vi "CRYDc volts out visa.vi"(10 "Volts":dbl step=0.0001 format="%.4f", 11 "COM port (0=COM1, etc.)":i32) -> (0 "error":bool)   [LabVIEW 2013]
panel:
  in  "VISA session (for class)":refnum<visa-resource-name>
  out "number":u16=28671 format="%.0x"
  out "error code":i32
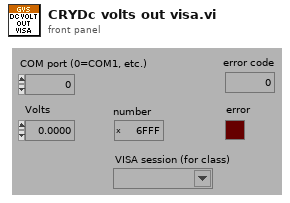
[diagram p1: front panel]
types:
  T1 = enum16{"noop", "clear DTR", "set DTR", "clear RTS", "set RTS", "set DTR protocol", "clr DTR protocol", "noop2"}
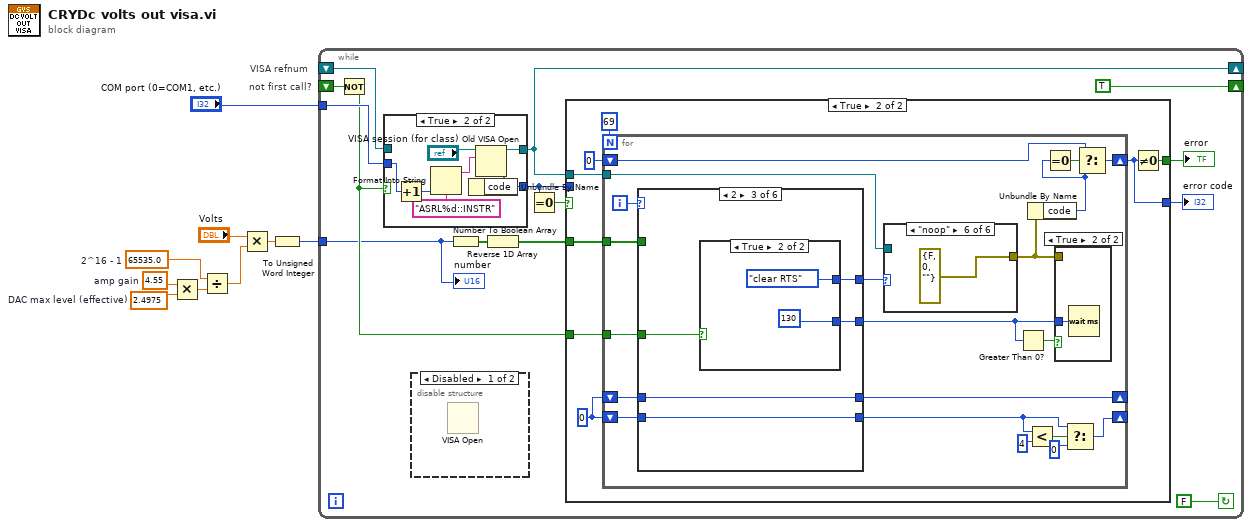
[diagram p0: block diagram]
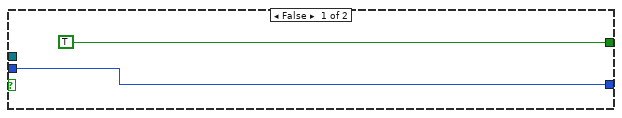
[diagram p3: hidden frame]
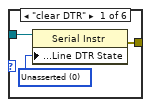
[diagram p4: hidden frame]
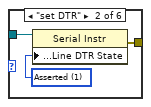
[diagram p5: hidden frame]
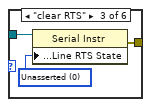
[diagram p6: hidden frame]
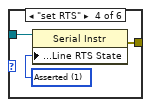
[diagram p7: hidden frame]
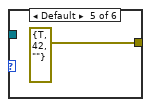
[diagram p8: hidden frame]
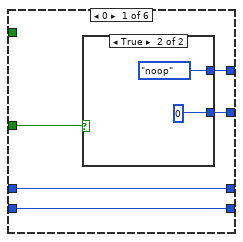
[diagram p10: hidden frame]
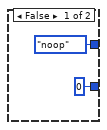
[diagram p11: hidden frame]
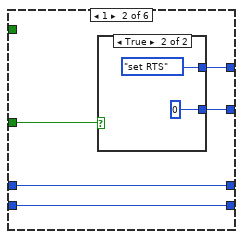
[diagram p12: hidden frame]
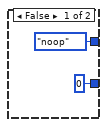
[diagram p13: hidden frame]
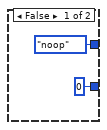
[diagram p14: hidden frame]
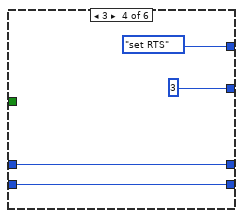
[diagram p15: hidden frame]
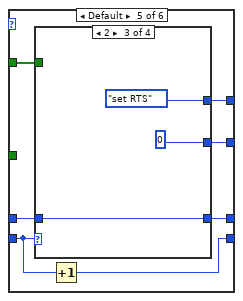
[diagram p16: hidden frame]
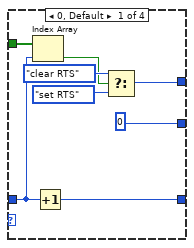
[diagram p17: hidden frame]
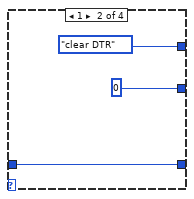
[diagram p18: hidden frame]
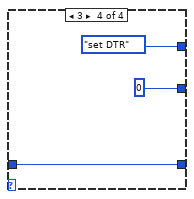
[diagram p19: hidden frame]
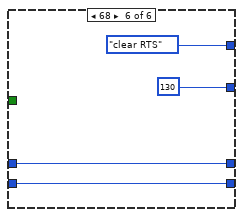
[diagram p20: hidden frame]
diagram:
  w5 = 2.4975  # DAC max level (effective)
  w7 = 65535.0  # 2^16 - 1
  w6 = 4.55  # amp gain
  # "VISA refnum"
  # "not first call?"
  n1 = Multiply(x=w6, y=w5) -> (x*y=w8:dbl)
  n2 = Divide(x=w7, y=w8) -> (x/y=w3:dbl)
  n3 = Multiply(x="Volts", y=w3) -> (x*y=w2:dbl)
  n4 = To Unsigned Word Integer(number=w2) -> (unsigned 16bit integer=w1:u16)
  n5 = while {
    tunnel: "COM port (0=COM1, etc.)" -> [w21]
    shift-right: [TRUE] -> _
    shift-left: _ -> [w19]
    tunnel: w1 -> [w17]
    shift-right: [w11] -> _
    shift-left: _ -> [w12]
    stop <- FALSE continue-if-true
    n6 = Not(x=w19) -> (.not. x?=w18:bool)
    n7 = case shown="True" w18 {
      tunnel: w21 -> [_ w135]
      tunnel: [0 ("error code") w130] -> w13
      tunnel: [w128 w132] -> w11
      tunnel: w12 -> [w128 _]
      frame False {
      }
      frame True {
        n8 = Increment(x=w135) -> (x+1=w134:i32)
        n9 = Format Into String(format string="ASRL%d::INSTR", w134) -> (resulting string=w136:string)  [unwired: 2 in, 1 out]
        n10 = Old VISA Open(10:w136, 11:"VISA session (for class)") -> (0:w131:errorcluster, 3:w132:refnum<visa-resource-name>)  [unwired: 1 in, 2 out]
        n11 = Unbundle By Name(w131) -> ("code"=w130:i32)
      }
    }
    n12 = disable-structure shown="Disabled" {
      frame Disabled {
        n13 = VISA Open() -> ()  [unwired: 5 in, 2 out]
      }
      frame Enabled {
      }
    }
    n14 = Number To Boolean Array(number=w17) -> (Boolean array=w23:bool[])
    n15 = Reverse 1D Array(array=w23) -> (reversed array=w22:bool[])
    n16 = Equal To 0?(x=w13) -> (x = 0?=w16:bool)
    n17 = case shown="True" w16 {
      tunnel: w22 -> [_ w33]
      tunnel: w18 -> [_ w30]
      tunnel: [TRUE w28] -> w15
      tunnel: [w24 w27] -> w14
      tunnel: w13 -> [w24 _]
      tunnel: w11 -> [_ w26]
      frame False {
      }
      frame True {
        w32 = 0
        n18 = for {
          N: 69 -> [_]
          tunnel: w33 -> [w52]
          shift-right: [w46] -> _
          shift-left: w32 -> [w51]
          shift-right: [w44] -> _
          shift-left: w32 -> [w45]
          tunnel: w30 -> [w43]
          shift-right: [w38] -> w27
          shift-left: 0 ("error code") -> [w40]
          tunnel: w26 -> [w34]
          i -> [w53]
          n19 = case shown="2" w53 {
            tunnel: [w73 w82 w91 T1."set RTS" ("function") w102 T1."clear RTS" ("function")] -> w37
            tunnel: [w72 w81 w90 u32 3 ("milliseconds to wait") w101 u32 130 ("milliseconds to wait")] -> w42
            tunnel: w52 -> [_ _ _ _ w103 _]
            tunnel: w51 -> [w71 w80 w89 w97 w105 w124]
            tunnel: [w71 w80 w89 w97 w106 w124] -> w47
            tunnel: w45 -> [w70 w79 w88 w96 w104 w125]
            tunnel: [w70 w79 w88 w96 w100 w125] -> w44
            tunnel: w43 -> [w69 w78 w87 _ _ _]
            frame 0 {
              n20 = case shown="True" w69 {
                tunnel: [T1."noop" ("function") T1."noop" ("function")] -> w73
                tunnel: [u32 0 ("milliseconds to wait") u32 0 ("milliseconds to wait")] -> w72
                frame False {
                }
                frame True {
                }
              }
            }
            frame 1 {
              n21 = case shown="True" w78 {
                tunnel: [T1."noop" ("function") T1."set RTS" ("function")] -> w82
                tunnel: [u32 0 ("milliseconds to wait") u32 0 ("milliseconds to wait")] -> w81
                frame False {
                }
                frame True {
                }
              }
            }
            frame 2 {
              n22 = case shown="True" w87 {
                tunnel: [T1."noop" ("function") T1."clear RTS" ("function")] -> w91
                tunnel: [u32 0 ("milliseconds to wait") u32 130 ("milliseconds to wait")] -> w90
                frame False {
                }
                frame True {
                }
              }
            }
            frame 3 {
            }
            frame Default {
              n23 = case shown="2" w105 {
                tunnel: w104 -> [w108 w115 w118 w121]
                tunnel: w103 -> [w114 _ _ _]
                tunnel: [w113 T1."clear DTR" ("function") T1."set RTS" ("function") T1."set DTR" ("function")] -> w102
                tunnel: [u32 0 ("milliseconds to wait") u32 0 ("milliseconds to wait") u32 0 ("milliseconds to wait") u32 0 ("milliseconds to wait")] -> w101
                tunnel: [w107 w115 w118 w121] -> w100
                frame 0, Default {
                  n24 = Index Array(array=w114, index=w108) -> (element=w110:bool)
                  n25 = Increment(x=w108) -> (x+1=w107:i32)
                  n26 = Select(t=T1."clear RTS" ("function"), s=w110, f=T1."set RTS" ("function")) -> (s? t:f=w113:T1)
                }
                frame 1 {
                }
                frame 2 {
                }
                frame 3 {
                }
              }
              n27 = Increment(x=w105) -> (x+1=w106:i32)
            }
            frame 68 {
            }
          }
          n28 = case shown="\"noop\"" w37 {
            tunnel: [w55 w58 w61 w64 errorcluster {"status"=TRUE, "code"=42, "source"=""} ("error out") errorcluster {"status"=FALSE, "code"=0, "source"=""} ("error out")] -> w35
            tunnel: w34 -> [w54 w57 w60 w63 _ _]
            frame "clear DTR" {
              w56 = i16 0 items=["Unknown"=-1, "Unasserted"=0, "Asserted"=1] ("Modem Line Settings:Line DTR State")
              n29 = property class="Serial Instr"(reference=w54, "Serial Settings:Modem Line Settings:Line DTR State"=w56) -> (error out=w55:errorcluster)  [unwired: 1 in, 1 out]
            }
            frame "set DTR" {
              w59 = i16 1 items=["Unknown"=-1, "Unasserted"=0, "Asserted"=1] ("Modem Line Settings:Line DTR State")
              n30 = property class="Serial Instr"(reference=w57, "Serial Settings:Modem Line Settings:Line DTR State"=w59) -> (error out=w58:errorcluster)  [unwired: 1 in, 1 out]
            }
            frame "clear RTS" {
              w62 = i16 0 items=["Unknown"=-1, "Unasserted"=0, "Asserted"=1] ("Modem Line Settings:Line DTR State")
              n31 = property class="Serial Instr"(reference=w60, "Serial Settings:Modem Line Settings:Line RTS State"=w62) -> (error out=w61:errorcluster)  [unwired: 1 in, 1 out]
            }
            frame "set RTS" {
              w65 = i16 1 items=["Unknown"=-1, "Unasserted"=0, "Asserted"=1] ("Modem Line Settings:Line DTR State")
              n32 = property class="Serial Instr"(reference=w63, "Serial Settings:Modem Line Settings:Line RTS State"=w65) -> (error out=w64:errorcluster)  [unwired: 1 in, 1 out]
            }
            frame Default {
            }
            frame "noop" {
            }
          }
          n33 = Greater Than 0?(x=w42) -> (x > 0?=w41:bool)
          n34 = Less?(x=w47, y=4) -> (x < y?=w49:bool)
          n35 = Unbundle By Name(w35) -> ("code"=w36:i32)
          n36 = Equal To 0?(x=w36) -> (x = 0?=w39:bool)
          n37 = case shown="True" w41 {
            tunnel: w42 -> [_ w68]
            tunnel: w35 -> [_ _]
            frame False {
            }
            frame True {
              n38 = Wait (ms)(milliseconds to wait=w68) -> ()  [unwired: 1 out]
            }
          }
          n39 = Select(t=w47, s=w49, f=0) -> (s? t:f=w46:i32)
          n40 = Select(t=w40, s=w39, f=w36) -> (s? t:f=w38:i32)
        }
        n41 = Not Equal To 0?(x=w27) -> (x != 0?=w28:bool)
      }
    }
    "error" <- w15
    "error code" <- w14
    "number" <- w17
  }
